vi "LJUD_eDI.vi"(8 "error in":errorcluster, 10 "Channel":i32, 11 "Handle In":i32) -> (0 "error out":errorcluster, 2 "State":i32, 3 "Handle Out":i32)   [LabVIEW 2018]
doc: "This is an easy function to read the\nstate of a single digital input. The\ndirection of the DIO is automatically\nset to input.\n\nSee Sections 4.2 and 4.3 of the device's\ndatasheet for more information."
uses:
  labjackud.dll
panel:
  # "This is an easy function to read the\nstate of a single digital input.  The\ndirection of the DIO is automatically\nset to input.\n\nSee Sections 4.2 and 4.3 of the device's\ndatasheet for more information."
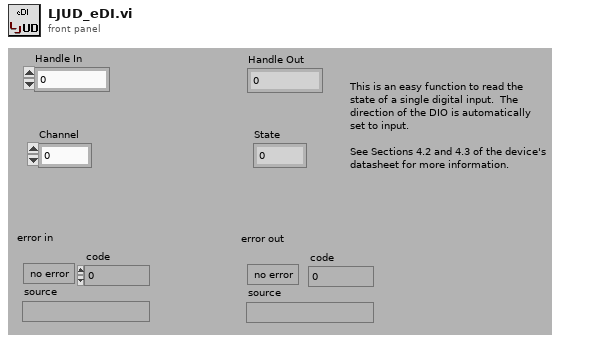
[diagram p1: front panel]
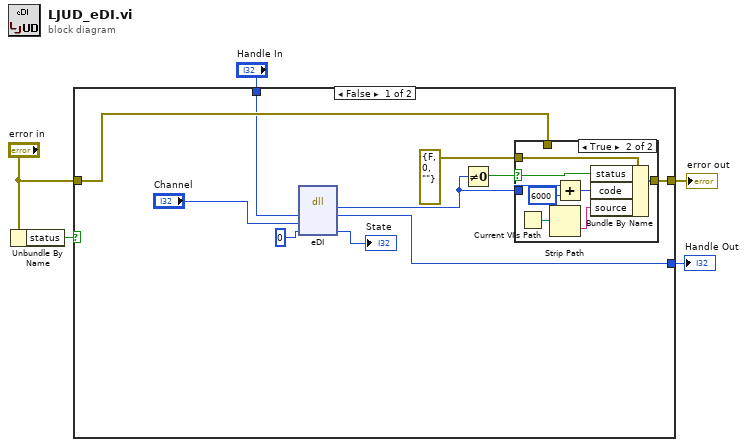
[diagram p0: block diagram]
diagram:
  n1 = Unbundle By Name("error in") -> ("status"=w4:bool)
  n2 = case shown="False" w4 {
    tunnel: [w12 w26] -> w5
    tunnel: "error in" -> [w11 w26]
    tunnel: "Handle In" -> [w7 w25]
    tunnel: [w6 w25] -> w1
    frame False {
      n3 = dll-call lib="labjackud.dll" fn="eDI"("Handle"=w7, "Channel"="Channel", "State"=0) -> (w13:i32, "Handle"=w6:i32, "State"=→"State":i32)  [unwired: 4 in, 2 out]
      n4 = Not Equal To 0?(x=w13) -> (x != 0?=w14:bool)
      n5 = case shown="True" w14 {
        selector: w14 -> [_ w23]
        tunnel: [w16 w24] -> w12
        tunnel: errorcluster {"status"=FALSE, "code"=0, "source"=""} ("error IO") -> [_ w22]
        tunnel: w13 -> [_ w18]
        tunnel: w11 -> [w16 _]
        frame False {
        }
        frame True {
          n6 = Current VI's Path() -> (path=w20:path)
          n7 = Strip Path(path=w20) -> (name=w21:string)  [unwired: 1 out]
          n8 = Add(x=w18, y=6000) -> (x+y=w19:i32)
          n9 = Bundle By Name(cluster=w22, "status"=w23, "code"=w19, "source"=w21) -> (w24:errorcluster)
        }
      }
    }
    frame True {
    }
  }
  "error out" <- w5
  "Handle Out" <- w1
